vi "readGearedMotorEnc.vi"(6 "Reset Counter":bool, 7 "Reverse ENC?":bool, 8 "error in (no error)":errorcluster) -> (0 "error out":errorcluster, 2 "gearedMotorEncoder (deg)":dbl)   [LabVIEW 2019, in "SJCube_ElvisIII.lvlib"]
uses:
  SJCube_ElvisIII.lvlib
  <vilib>/myRIO/Common/Instrument Driver Framework/myRIO v1.0/Encoder/typedefs/Encoder Count Direction Enum.ctl
  <vilib>/myRIO/Common/Instrument Driver Framework/myRIO v1.0/Encoder/typedefs/Encoder Signal Mode.ctl
  <vilib>/myRIO/Common/Instrument Driver Framework/myRIO v1.0/Encoder/typedefs/Encoder Channels Enum.ctl
  <vilib>/myRIO/Common/Instrument Driver Framework/Utilities/typedefs/Generic FPGA Reference.ctl
  <vilib>/myRIO/Common/Instrument Driver Framework/Utilities/typedefs/myRIO v1.0 Reference.ctl
  <vilib>/myRIO/Common/Instrument Driver Framework/Utilities/typedefs/Hardware Version Enum.ctl
  <vilib>/myRIO/Common/Instrument Driver Framework/Utilities/typedefs/myRIO Generic Hardware Reference.ctl
  <vilib>/myRIO/Instrument Drivers/Onboard IO/Encoder/typedefs/Encoder Reference.ctl
  <vilib>/myRIO/Instrument Drivers/Onboard IO/Encoder/Encoder.lvlib
  <vilib>/myRIO/Instrument Drivers/Onboard IO/Encoder/vis/Read.vi
  <vilib>/myRIO/Instrument Drivers/Onboard IO/Encoder/vis/myRIO Encoder Open.xnode
  <vilib>/myRIO/Common/Instrument Driver Framework/Utilities/vis/Is FPGA Ref Available.vi
  <vilib>/myRIO/Express VI/Onboard IO/Encoder/Encoder Express VI.xnode
  <vilib>/myRIO/Common/Instrument Driver Framework/ELVIS III v1.0/Encoder/vis/ELVIS III v1.1 Open Encoder.vi
  <vilib>/myRIO/Common/Instrument Driver Framework/ELVIS III v1.0/Encoder/vis/ELVIS III v1.0 Configure Encoder.vi
  <vilib>/myRIO/Common/Instrument Driver Framework/myRIO v1.0/Encoder/typedefs/Encoder Configuration v1.0.ctl
  <vilib>/userDefined/High Color/nirio_resource_hc.ctl
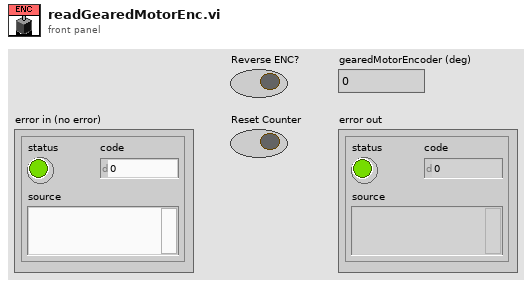
[diagram p1: front panel]
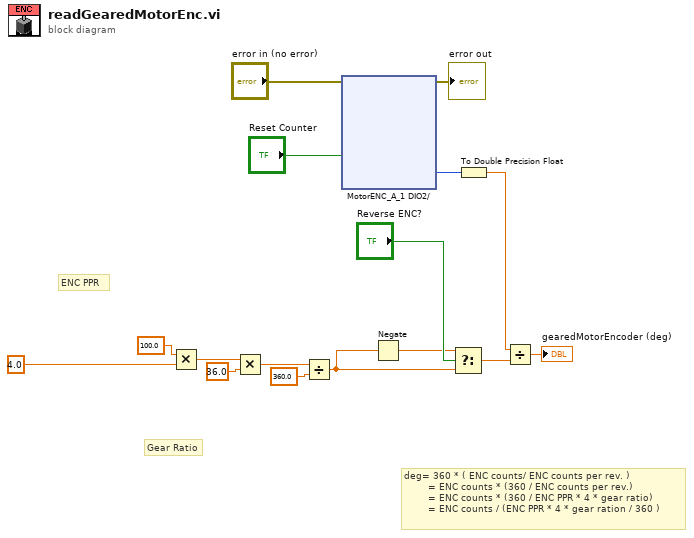
[diagram p0: block diagram]
diagram:
  # "Gear Ratio"
  # "ENC PPR"
  # "deg= 360 * ( ENC counts/ ENC counts per rev. )\n        = ENC counts * (360 / ENC counts per rev.)\n        = ENC counts * (360 / ENC PPR * 4 * gear ratio)\n        = ENC counts / (ENC PPR * 4 * gear ration / 360 )"
  n1 = Multiply(x=100.0 ("y"), y=4.0) -> (x*y=w6:dbl)
  n2 = Multiply(x=w6, y=36.0) -> (x*y=w4:dbl)
  n3 = Divide(x=w4, y=360.0) -> (x/y=w1:dbl)
  n4 = xnode "MotorENC_A_1 DIO2/"("Reset Counter"="Reset Counter", "error in (no error)"="error in (no error)") -> ("Counter Value"=w13:i32, "error out"=→"error out":errorcluster)  [unwired: 2 out]
  n5 = Negate(x=w1) -> (-x=w2:dbl)
  n6 = Select(t=w2, s="Reverse ENC?", f=w1) -> (s? t:f=w9:dbl)
  n7 = To Double Precision Float(number=w13) -> (double precision float=w12:dbl)
  n8 = Divide(x=w12, y=w9) -> (x/y=→"gearedMotorEncoder (deg)":dbl)
